vi "SetVesselCluster.vi"(8 "error in (no error)":errorcluster, 10 "Vessel Cluster":T1, 11 "Image in":refnum<class "Image.lvclass">) -> (0 "error out":errorcluster, 3 "Image out":refnum<class "Image.lvclass">)   [LabVIEW 2011, in "Image.lvclass"]
uses:
  Image.lvclass
  Image.lvclass/Image.ctl
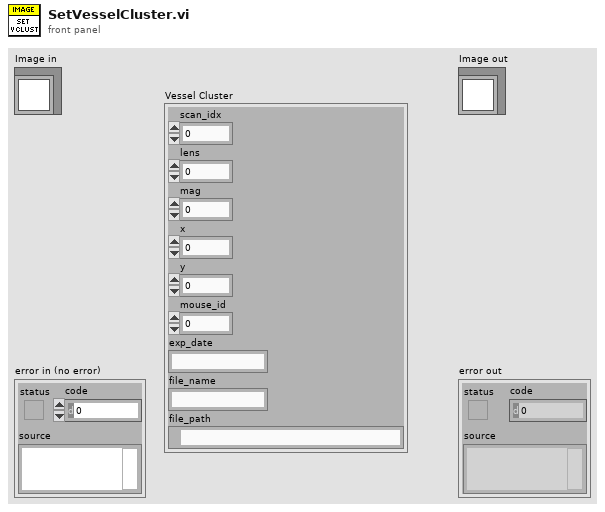
[diagram p1: front panel]
types:
  T1 = cluster{"scan_idx":i32, "lens":i32, "mag":dbl, "x":dbl, "y":dbl, "mouse_id":i32, "exp_date":string, "file_name":string, "file_path":path}
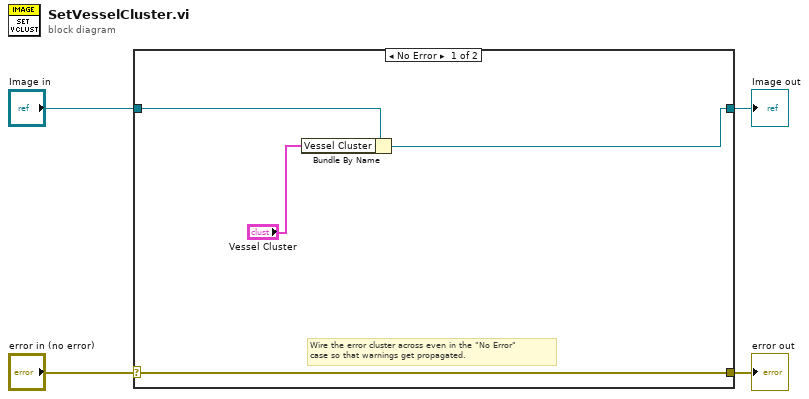
[diagram p0: block diagram]
diagram:
  n1 = case shown="No Error" "error in (no error)" {
    selector: "error in (no error)" -> [w8 w10]
    tunnel: [w8 w10] -> w3
    tunnel: [w6 w9] -> w1
    tunnel: "Image in" -> [w7 w9]
    frame No Error {
      # "Wire the error cluster across even in the \"No Error\"\ncase so that warnings get propagated."
      n2 = Bundle By Name(cluster=w7, "Vessel Cluster"="Vessel Cluster") -> (w6:refnum<class "Image.lvclass">)
    }
    frame Error {
    }
  }
  "error out" <- w3
  "Image out" <- w1
